vi "CreateXmlFromReadings.vi"(8 "error in":errorcluster) -> (0 "error out":errorcluster, 3 "xml string":string)   [LabVIEW 2020]
uses:
  ProcessData.ctl
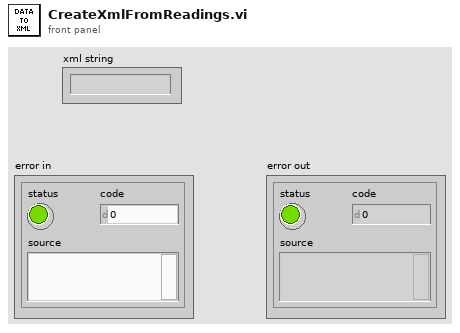
[diagram p1: front panel]
types:
  T1 = typedef "ProcessData.ctl" = cluster{"Level":dbl, "Aeration":bool, "Feed":bool, "Mixer":bool, "Overflow":bool, "Recycle":bool, "Substrate":bool, "CO2":dbl, "Mixing":dbl, "pH":dbl, "Temperature":dbl, "Redox":dbl, "Turbidity":dbl, "Oxygen":dbl, "Flow":dbl}
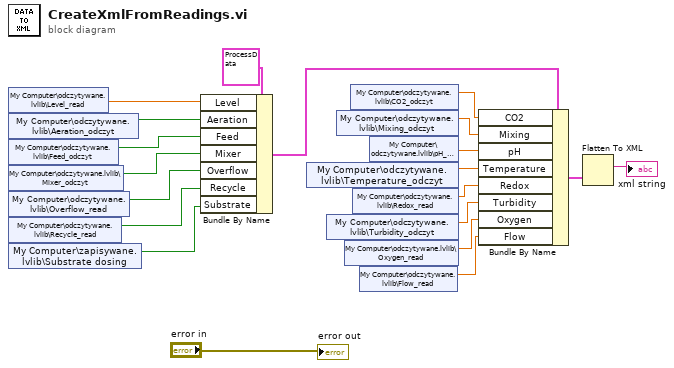
[diagram p0: block diagram]
diagram:
  n1 = shared-variable "My Computer\\odczytywane.lvlib\\Level_read"() -> (w19:dbl)  [unwired: 1 in, 1 out]
  n2 = shared-variable "My Computer\\odczytywane.lvlib\\Aeration_odczyt"() -> (w16:bool)  [unwired: 1 in, 1 out]
  n3 = shared-variable "My Computer\\odczytywane.lvlib\\Feed_odczyt"() -> (w15:bool)  [unwired: 1 in, 1 out]
  n4 = shared-variable "My Computer\\odczytywane.lvlib\\Mixer_odczyt"() -> (w14:bool)  [unwired: 1 in, 1 out]
  n5 = shared-variable "My Computer\\odczytywane.lvlib\\Overflow_read"() -> (w13:bool)  [unwired: 1 in, 1 out]
  n6 = shared-variable "My Computer\\odczytywane.lvlib\\Recycle_read"() -> (w12:bool)  [unwired: 1 in, 1 out]
  n7 = shared-variable "My Computer\\zapisywane.lvlib\\Substrate dosing"() -> (w11:bool)  [unwired: 1 in, 1 out]
  n8 = Bundle By Name(cluster=T1 {"Level"=0.0, "Aeration"=FALSE, "Feed"=FALSE, "Mixer"=FALSE, "Overflow"=FALSE, "Recycle"=FALSE, "Substrate"=FALSE, "CO2"=0.0, "Mixing"=0.0, "pH"=0.0, "Temperature"=0.0, "Redox"=0.0, "Turbidity"=0.0, "Oxygen"=0.0, "Flow"=0.0} ("Cluster"), "Level"=w19, "Aeration"=w16, "Feed"=w15, "Mixer"=w14, "Overflow"=w13, "Recycle"=w12, "Substrate"=w11) -> (w10:T1)
  n9 = shared-variable "My Computer\\odczytywane.lvlib\\Temperature_odczyt"() -> (w5:dbl)  [unwired: 1 in, 1 out]
  n10 = shared-variable "My Computer\\odczytywane.lvlib\\Turbidity_odczyt"() -> (w3:dbl)  [unwired: 1 in, 1 out]
  n11 = shared-variable "My Computer\\odczytywane.lvlib\\Mixing_odczyt"() -> (w7:dbl)  [unwired: 1 in, 1 out]
  n12 = shared-variable "My Computer\\odczytywane.lvlib\\Oxygen_read"() -> (w9:dbl)  [unwired: 1 in, 1 out]
  n13 = shared-variable "My Computer\\odczytywane.lvlib\\CO2_odczyt"() -> (w8:dbl)  [unwired: 1 in, 1 out]
  n14 = shared-variable "My Computer\\odczytywane.lvlib\\Redox_read"() -> (w4:dbl)  [unwired: 1 in, 1 out]
  n15 = shared-variable "My Computer\\odczytywane.lvlib\\Flow_read"() -> (w1:dbl)  [unwired: 1 in, 1 out]
  n16 = shared-variable "My Computer\\odczytywane.lvlib\\pH_read"() -> (w6:dbl)  [unwired: 1 in, 1 out]
  n17 = Bundle By Name(cluster=w10, "CO2"=w8, "Mixing"=w7, "pH"=w6, "Temperature"=w5, "Redox"=w4, "Turbidity"=w3, "Oxygen"=w9, "Flow"=w1) -> (w2:T1)
  n18 = Flatten To XML(6:w2) -> (2:→"xml string":string)
  "error out" <- "error in"
